vi "Measurement Logic.vi"() -> ()   [LabVIEW 2021, in "audio_acMeasurement.lvlib"]
uses:
  audio_acMeasurement.lvlib
  <resource>/objmgr/daqmx.rc
  <vilib>/PDM Acquisition Toolkit/host/API/PDM Acquisition Toolkit.lvlib
  <vilib>/PDM Acquisition Toolkit/host/Classes/Tasks/PCM Input/PCM Input Task.lvclass
  <vilib>/PDM Acquisition Toolkit/host/Classes/Tasks/PCM Input/Controls/DVR PCM Input Task.ctl
  <vilib>/DAQmx/configure/timing.llb/DAQmx Timing (Sample Clock).vi
  <vilib>/DAQmx/create/channels.llb/DAQmx Create Channel (AO-Voltage-Basic).vi
  <vilib>/DAQmx/create/channels.llb/DAQmx Create Channel (AO-FuncGen).vi
  <vilib>/PDM Acquisition Toolkit/host/API/Public/Read/Read PCM Input Waveform.vi
  <vilib>/PDM Acquisition Toolkit/host/API/Public/Start/Start PCM Input Task.vi
  <vilib>/PDM Acquisition Toolkit/host/API/Public/Clear/Clear PCM Input Task.vi
  shared/controls/Settings.ctl
  shared/controls/Protocol Configurations.ctl
  Measurement Configuration.ctl
  <vilib>/MeasurementLink/MeasurementLink Measurement Server/Classes/MeasurementContext/MeasurementContext.lvclass
  Measurement Results.ctl
panel:
  out "Measurement Results":T1
  out "Measurement Context out":refnum<class "MeasurementContext.lvclass">
  in  "Measurement Context":refnum<class "MeasurementContext.lvclass">
  in  "Measurement Configuration":T2={"Band start"=20.0, "Band stop"=20000.0, "Weighting filter"=0, "Full scale range"=3.16, "Analog source resource name"="", "Frequency"=1000.0, "Amplitude"=-1.0, "Protocol capture resource name"="", "Protocol capture channel"="0L", "JSON file"="", "Clock rate"=12288000, "Number of words"=19200, "Sensitivity"=0.34762} {"Clock rate" format="%#.0f"}
  out "error out":errorcluster
  in  "error in":errorcluster
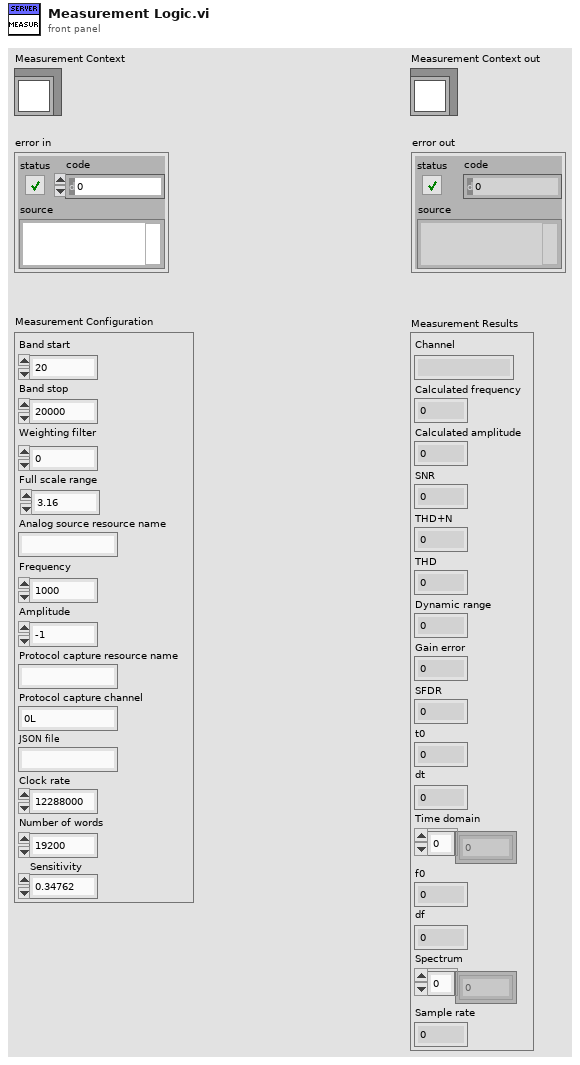
[diagram p1: front panel]
types:
  T1 = typedef "audio_acMeasurement.lvlib/Measurement Results.ctl" = cluster{"Channel":string, "Calculated frequency":dbl, "Calculated amplitude":dbl, "SNR":dbl, "THD+N":dbl, "THD":dbl, "Dynamic range":dbl, "Gain error":dbl, "SFDR":dbl, "t0":dbl, "dt":dbl, "Time domain":dbl[], "f0":dbl, "df":dbl, "Spectrum":dbl[], "Sample rate":u32}
  T2 = typedef "audio_acMeasurement.lvlib/Measurement Configuration.ctl" = cluster{"Band start":dbl, "Band stop":dbl, "Weighting filter":u16, "Full scale range":dbl, "Analog source resource name":string, "Frequency":dbl, "Amplitude":dbl, "Protocol capture resource name":string, "Protocol capture channel":string, "JSON file":string, "Clock rate":u32, "Number of words":u32, "Sensitivity":dbl}
  T3 = typedef "PDM Acquisition Class Library.lvlib/PCM Input Task.lvclass/DVR PCM Input Task.ctl" = refnum<data-value>
  T4 = typedef "Settings.ctl" = cluster{"Frame_Sync_Edge_for_Channel 0":i32, "Channel_Count_Per_Frame":i32, "Channel_Length":i32, "Bit_Depth":i32, "Channel_0_Offset":i32, "Endianness":i32, "Data_Justification":i32, "Frame_Length":i32, "Frame_Sync_Pulse_Width":i32, "Bit_Clock_Edge_Sync":i32}
  T5 = cluster{"DSG Session":refnum<k21>, "PCM input task out":T3, "Calculated sample rate":u32, "Settings":T4}
  T6 = typedef "Protocol Configurations.ctl" = cluster{"Protocol capture resource name":string, "Protocol capture channel":string, "Clock rate":u32, "Number of words":u32, "Sensitivity":dbl, "Settings":T4}
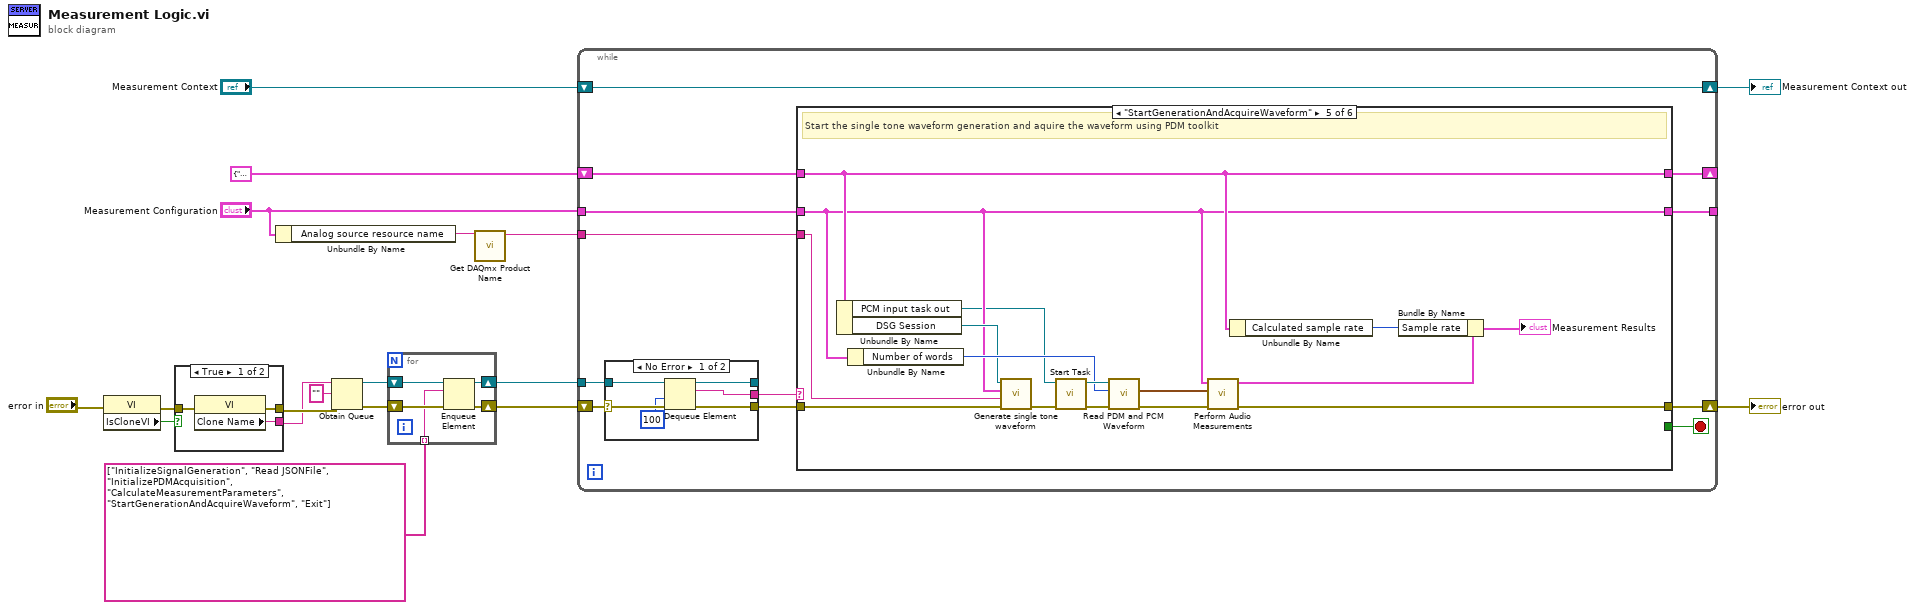
[diagram p0: block diagram]
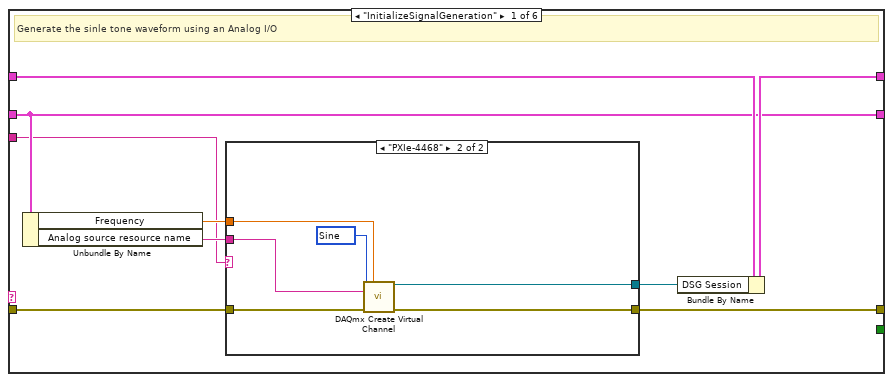
[diagram p2: hidden frame]
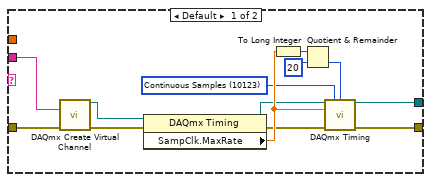
[diagram p3: hidden frame]
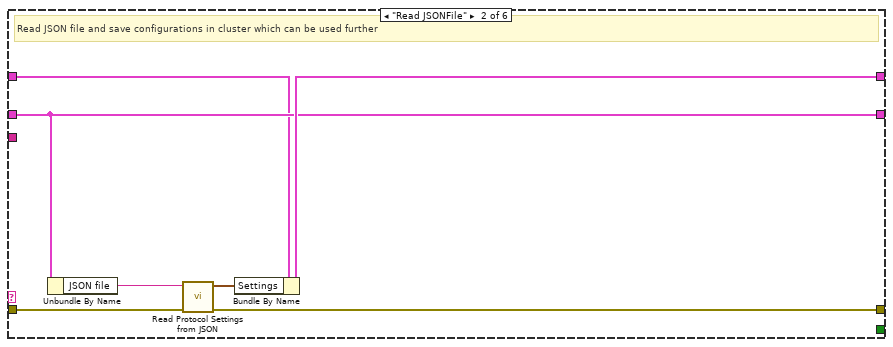
[diagram p4: hidden frame]
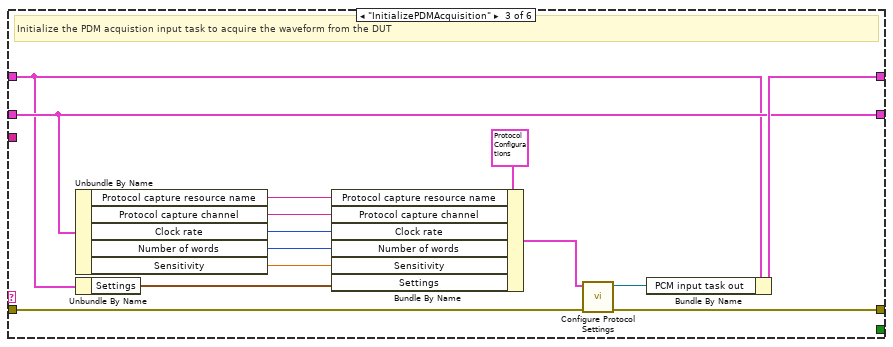
[diagram p5: hidden frame]
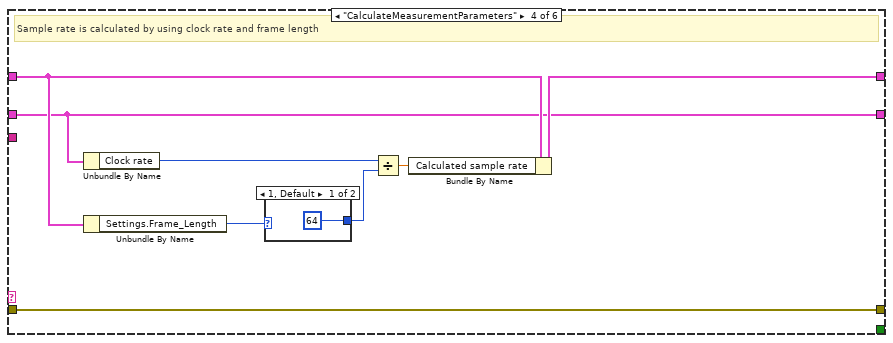
[diagram p6: hidden frame]
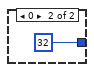
[diagram p7: hidden frame]
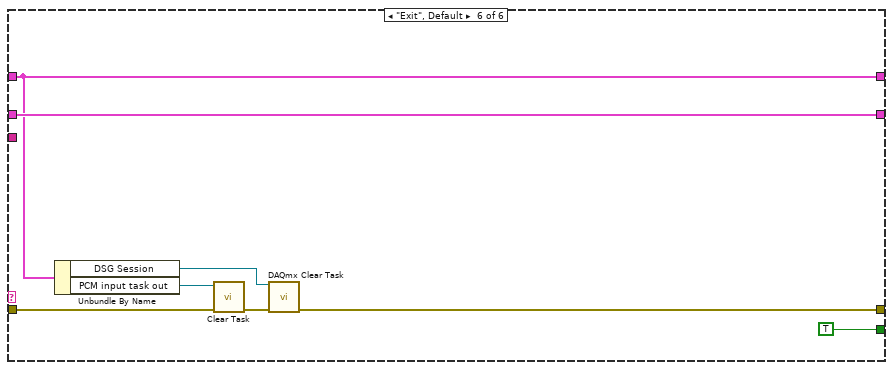
[diagram p8: hidden frame]
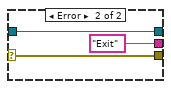
[diagram p9: hidden frame]
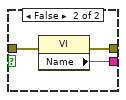
[diagram p10: hidden frame]
diagram:
  n1 = property class="VI"(error in="error in") -> (error out=w14:errorcluster, "IsCloneVI"=w15:bool)  [unwired: 1 in, 1 out]
  n2 = case shown="True" w15 {
    tunnel: [w21 w24] -> w13
    tunnel: [w20 w23] -> w12
    tunnel: w14 -> [w19 w22]
    frame True {
      n3 = property class="VI"(error in=w19) -> (error out=w21:errorcluster, "Clone Name"=w20:string)  [unwired: 1 in, 1 out]
    }
    frame False {
      n4 = property class="VI"(error in=w22) -> (error out=w24:errorcluster, "Name"=w23:string)  [unwired: 1 in, 1 out]
    }
  }
  n5 = Unbundle By Name("Measurement Configuration") -> ("Analog source resource name"=w5:string)
  n6 = Obtain Queue(name (unnamed)=w12, element data type="", error in (no error)=w13) -> (queue out=w17:refnum<queue>, error out=w11:errorcluster)  [unwired: 2 in, 1 out]
  n7 = for {
    shift-right: [w27] -> w10
    shift-left: w17 -> [w29]
    shift-right: [w26] -> w9
    shift-left: w11 -> [w28]
    tunnel: string[] ["InitializeSignalGeneration", "Read JSONFile", "InitializePDMAcquisition", "CalculateMeasurementParameters", "StartGenerationAndAcquireWaveform", "Exit"] ("Step sequence") -> [w25] mode=indexing
    n8 = Enqueue Element(queue=w29, element=w25, error in (no error)=w28) -> (queue out=w27:refnum<queue>, error out=w26:errorcluster)  [unwired: 1 in, 1 out]
  }
  n9 = call "Get DAQmx Product Name.vi"("DAQmx resource name"=w5) -> ("DAQmx product type"=w3:string)  [unwired: 10 in]
  n10 = while {
    tunnel: w10 -> [w41]
    shift-right: [w39] -> w2
    shift-left: w9 -> [w38]
    shift-right: [w34] -> w6
    shift-left: "Measurement Context" -> [w34]
    tunnel: "Measurement Configuration" -> [w35]
    tunnel: [w36] -> _
    shift-right: [w32] -> _
    shift-left: T5 {"DSG Session"="", "PCM input task out"=refnum, "Calculated sample rate"=0, "Settings"={"Frame_Sync_Edge_for_Channel 0"=0, "Channel_Count_Per_Frame"=0, "Channel_Length"=0, "Bit_Depth"=0, "Channel_0_Offset"=0, "Endianness"=0, "Data_Justification"=0, "Frame_Length"=0, "Frame_Sync_Pulse_Width"=0, "Bit_Clock_Edge_Sync"=0}} -> [w37]
    tunnel: w3 -> [w31]
    stop <- w33 stop-if-true
    n11 = case shown="No Error" w38 {
      selector: w38 -> [w128 w132]
      tunnel: w41 -> [w130 w131]
      tunnel: [w129 "Exit" ("t")] -> w30
      tunnel: [w127 w132] -> w40
      tunnel: [w125 w131] -> _
      frame No Error {
        n12 = Dequeue Element(queue=w130, timeout in ms (-1)=100, error in (no error)=w128) -> (queue out=w125:refnum<queue>, element=w129:string, error out=w127:errorcluster)  [unwired: 1 out]
      }
      frame Error {
      }
    }
    n13 = case shown="\"StartGenerationAndAcquireWaveform\"" w30 {
      tunnel: w40 -> [w49 w75 w89 w95 w113 w123]
      tunnel: [w48 w74 w81 w95 w108 w121] -> w39
      tunnel: w35 -> [w45 w72 w88 w91 w102 w124]
      tunnel: w37 -> [w47 w71 w79 w94 w103 w120]
      tunnel: [w46 w73 w90 w92 w103 w120] -> w32
      tunnel: [w45 w72 w88 w91 w102 w124] -> w36
      tunnel: [_ _ _ _ _ TRUE] -> w33
      tunnel: w31 -> [w43 _ _ _ w110 _]
      frame "InitializeSignalGeneration" {
        # "Generate the sinle tone waveform using an Analog I/O"
        n14 = Unbundle By Name(w45) -> ("Frequency"=w44:dbl, "Analog source resource name"=w50:string)
        n15 = case shown="\"PXIe-4468\"" w43 {
          tunnel: w50 -> [w63 w66]
          tunnel: w49 -> [w51 w69]
          tunnel: [w62 w68] -> w48
          tunnel: [w52 w67] -> w42
          tunnel: w44 -> [_ w64]
          frame Default {
            w53 = 10123 items=["Finite Samples"=10178, "Continuous Samples"=10123, "Hardware Timed Single Point"=12522] ("sample mode")
            n16 = call-poly <vilib>:"DAQmx Create Virtual Channel.vi"("physical channels"=w63, "error in"=w51) -> ("task out"=w61:refnum<k21>, "error out"=w60:errorcluster)  [unwired: 12 in]
            n17 = property class="DAQmx Timing"(reference=w61, error in=w60) -> (reference out=w56:refnum<k21>, error out=w57:errorcluster, "SampClk.MaxRate"=w58:dbl)
            n18 = To Long Integer(number=w58) -> (32bit integer=w54:i32)
            n19 = Quotient & Remainder(x=w54, y=20) -> (floor(x/y)=w59:i32)  [unwired: 1 out]
            n20 = call-poly <vilib>:"DAQmx Timing.vi"("task/channels in"=w56, "sample mode"=w53, "samples per channel"=w59, "rate"=w58, "error in"=w57) -> ("task out"=w52:refnum<k21>, "error out"=w62:errorcluster)  [unwired: 9 in]
          }
          frame "PXIe-4468" {
            w65 = 14751 items=["Sine"=14751, "Triangle"=14752, "Square"=14753, "Sawtooth"=14754] ("type")
            n21 = call-poly <vilib>:"DAQmx Create Virtual Channel.vi"("frequency"=w64, "physical channels"=w66, "type"=w65, "error in"=w69) -> ("task out"=w67:refnum<k21>, "error out"=w68:errorcluster)  [unwired: 10 in]
          }
        }
        n22 = Bundle By Name(cluster=w47, "DSG Session"=w42) -> (w46:T5)
      }
      frame "Read JSONFile" {
        # "Read JSON file and save configurations in cluster which can be used further"
        n23 = Unbundle By Name(w72) -> ("JSON file"=w76:string)
        n24 = call "Read Protocol Settings from JSON.vi"("error in"=w75, "JSON file"=w76) -> ("error out"=w74:errorcluster, "Settings"=w70:T4)  [unwired: 8 in]
        n25 = Bundle By Name(cluster=w71, "Settings"=w70) -> (w73:T5)
      }
      frame "InitializePDMAcquisition" {
        # "Initialize the PDM acquistion input task to acquire the waveform from the DUT"
        n26 = Unbundle By Name(w88) -> ("Protocol capture resource name"=w87:string, "Protocol capture channel"=w86:string, "Clock rate"=w85:u32, "Number of words"=w84:u32, "Sensitivity"=w83:dbl)
        n27 = Unbundle By Name(w79) -> ("Settings"=w78:T4)
        n28 = Bundle By Name(cluster=T6 {"Protocol capture resource name"="PXI1Slot7", "Protocol capture channel"="0L", "Clock rate"=12288000, "Number of words"=19200, "Sensitivity"=0.34762, "Settings"={"Frame_Sync_Edge_for_Channel 0"=0, "Channel_Count_Per_Frame"=0, "Channel_Length"=0, "Bit_Depth"=0, "Channel_0_Offset"=0, "Endianness"=0, "Data_Justification"=0, "Frame_Length"=0, "Frame_Sync_Pulse_Width"=0, "Bit_Clock_Edge_Sync"=0}} ("Protocol Configurations"), "Protocol capture resource name"=w87, "Protocol capture channel"=w86, "Clock rate"=w85, "Number of words"=w84, "Sensitivity"=w83, "Settings"=w78) -> (w80:T6)
        n29 = call "Configure Protocol Settings.vi"("error in (no error)"=w89, "Protocol Configurations"=w80) -> ("error out"=w81:errorcluster, "PCM input task out"=w82:T3)  [unwired: 8 in]
        n30 = Bundle By Name(cluster=w79, "PCM input task out"=w82) -> (w90:T5)
      }
      frame "CalculateMeasurementParameters" {
        # "Sample rate is calculated by using clock rate and frame length"
        n31 = Unbundle By Name(w91) -> ("Clock rate"=w98:u32)
        n32 = Unbundle By Name(w94) -> ("Settings.Frame_Length"=w93:i32)
        n33 = case shown="1, Default" w93 {
          tunnel: [64 32] -> w96
          frame 1, Default {
          }
          frame 0 {
          }
        }
        n34 = Divide(x=w98, y=w96) -> (x/y=w97:dbl)
        n35 = Bundle By Name(cluster=w94, "Calculated sample rate"=w97) -> (w92:T5)
      }
      frame "StartGenerationAndAcquireWaveform" {
        # "Start the single tone waveform generation and aquire the waveform using PDM toolkit"
        n36 = Unbundle By Name(w103) -> ("PCM input task out"=w101:T3, "DSG Session"=w111:refnum<k21>)
        n37 = Unbundle By Name(w102) -> ("Number of words"=w112:u32)
        n38 = call "Generate single tone waveform.vi"("error in (no error)"=w113, "DAQmx product type"=w110, "Measurement Configuration"=w102, "DSG task in"=w111) -> ("error out"=w114:errorcluster)  [unwired: 6 in, 1 out]
        n39 = call-poly <vilib>:"Start Task.vi"("error in"=w114, "PCM input task in"=w101) -> ("error out"=w116:errorcluster, "PCM input task out"=w115:T3)  [unwired: 8 in]
        n40 = call-poly <vilib>:"Read PDM and PCM Waveform.vi"("error in"=w116, "words per channel"=w112, "PCM input task In"=w115) -> ("error out"=w109:errorcluster, "PCM waveforms"=w107:waveform(dbl)[])  [unwired: 5 in, 2 out]
        n41 = call "Perform Audio Measurements.vi"("Measurement Configuration"=w102, "I2S waveforms"=w107, "error in (no error)"=w109) -> ("Measurement Results"=w106:T1, "error out"=w108:errorcluster)  [unwired: 6 in]
        n42 = Unbundle By Name(w103) -> ("Calculated sample rate"=w105:u32)
        n43 = Bundle By Name(cluster=w106, "Sample rate"=w105) -> (→"Measurement Results":T1)
      }
      frame "Exit", Default {
        n44 = Unbundle By Name(w120) -> ("DSG Session"=w119:refnum<k21>, "PCM input task out"=w117:T3)
        n45 = call-poly <vilib>:"Clear Task.vi"("error in"=w123, "PCM input task in"=w117) -> ("error out"=w122:errorcluster)  [unwired: 9 in]
        n46 = call <vilib>:"DAQmx Clear Task.vi"("task in"=w119, "error in"=w122) -> ("error out"=w121:errorcluster)  [unwired: 13 in]
      }
    }
  }
  "error out" <- w2
  "Measurement Context out" <- w6
